vi "Write Connection Configuration.vi"(8 "error in (no error)":errorcluster, 10 "Client Connection Configuration":T1, 11 "OPC UA Client configuration in":refnum<class "OPC UA Client configuration.lvclass">) -> (0 "error out":errorcluster, 3 "OPC UA Client configuration out":refnum<class "OPC UA Client configuration.lvclass">)   [LabVIEW 2014, in "OPC UA Client configuration.lvclass"]
uses:
  OPC UA Client configuration.lvclass
  Client Connection Configuration.ctl
  OPC UA Client configuration.lvclass/OPC UA Client configuration.ctl
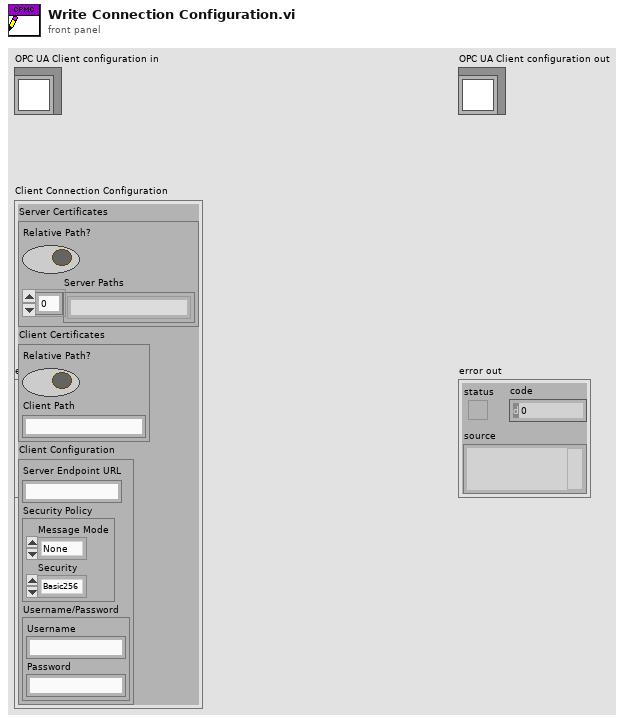
[diagram p1: front panel]
types:
  T1 = typedef "OPC UA Client configuration.lvclass/Client Connection Configuration.ctl" = cluster{"Server Certificates":cluster{"Relative Path?":bool, "Server Paths":string[]}, "Client Certificates":cluster{"Relative Path?":bool, "Client Path":string}, "Client Configuration":cluster{"Server Endpoint URL":string, "Security Policy":cluster{"Message Mode":enum16{"None", "Sign", "Sign and Encrypt"}, "Security":enum16{"Basic256", "Basic128Rsa15"}}, "Username/Password":cluster{"Username":string, "Password":string}}}
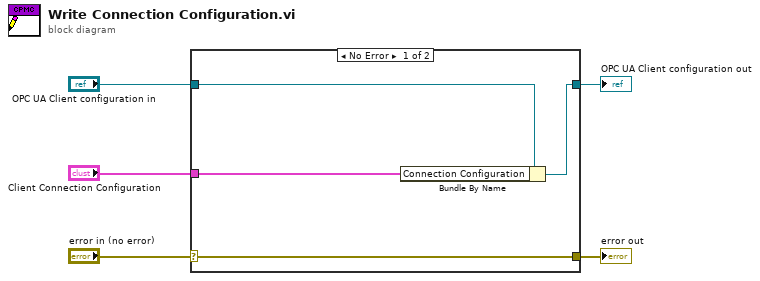
[diagram p0: block diagram]
diagram:
  n1 = case shown="No Error" "error in (no error)" {
    selector: "error in (no error)" -> [w9 w10]
    tunnel: [w9 w10] -> w4
    tunnel: [w7 w11] -> w2
    tunnel: "OPC UA Client configuration in" -> [w8 w11]
    tunnel: "Client Connection Configuration" -> [w6 _]
    frame No Error {
      n2 = Bundle By Name(cluster=w8, "Connection Configuration"=w6) -> (w7:refnum<class "OPC UA Client configuration.lvclass">)
    }
    frame Error {
    }
  }
  "error out" <- w4
  "OPC UA Client configuration out" <- w2
